vi "Get Calculated Tournament Stats.vi"(11 "Tournament Stats":T2) -> (3 "Calculated Tournament Stats":T1)   [LabVIEW 2021]
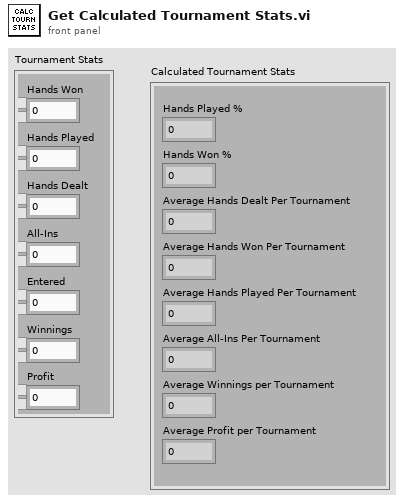
[diagram p1: front panel]
types:
  T1 = cluster{"Hands Played %":dbl, "Hands Won %":dbl, "Average Hands Dealt Per Tournament":dbl, "Average Hands Won Per Tournament":dbl, "Average Hands Played Per Tournament":dbl, "Average All-Ins Per Tournament":dbl, "Average Winnings per Tournament":dbl, "Average Profit per Tournament":dbl}
  T2 = cluster{"Hands Won":u32, "Hands Played":u32, "Hands Dealt":u32, "All-Ins":u32, "Entered":u32, "Winnings":dbl, "Profit":dbl}
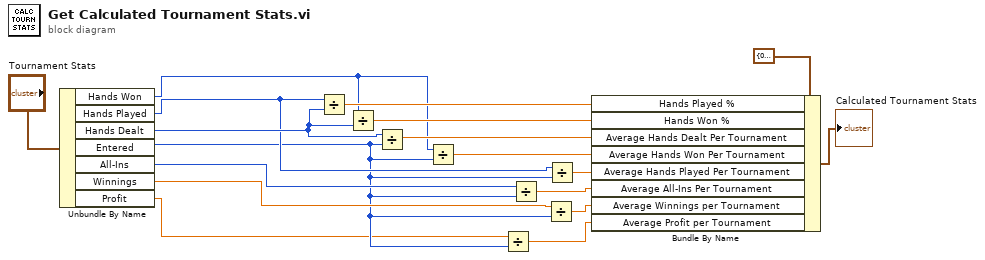
[diagram p0: block diagram]
diagram:
  n1 = Unbundle By Name("Tournament Stats") -> ("Hands Won"=w13:u32, "Hands Played"=w8:u32, "Hands Dealt"=w14:u32, "Entered"=w2:u32, "All-Ins"=w6:u32, "Winnings"=w4:dbl, "Profit"=w1:dbl)
  n2 = Divide(x=w8, y=w14) -> (x/y=w17:dbl)
  n3 = Divide(x=w13, y=w14) -> (x/y=w16:dbl)
  n4 = Divide(x=w14, y=w2) -> (x/y=w15:dbl)
  n5 = Divide(x=w13, y=w2) -> (x/y=w12:dbl)
  n6 = Divide(x=w1, y=w2) -> (x/y=w3:dbl)
  n7 = Divide(x=w6, y=w2) -> (x/y=w7:dbl)
  n8 = Divide(x=w4, y=w2) -> (x/y=w5:dbl)
  n9 = Divide(x=w8, y=w2) -> (x/y=w9:dbl)
  n10 = Bundle By Name(cluster=T1 {"Hands Played %"=0.0, "Hands Won %"=0.0, "Average Hands Dealt Per Tournament"=0.0, "Average Hands Won Per Tournament"=0.0, "Average Hands Played Per Tournament"=0.0, "Average All-Ins Per Tournament"=0.0, "Average Winnings per Tournament"=0.0, "Average Profit per Tournament"=0.0} ("Calculated Tournament Stats"), "Hands Played %"=w17, "Hands Won %"=w16, "Average Hands Dealt Per Tournament"=w15, "Average Hands Won Per Tournament"=w12, "Average Hands Played Per Tournament"=w9, "Average All-Ins Per Tournament"=w7, "Average Winnings per Tournament"=w5, "Average Profit per Tournament"=w3) -> (→"Calculated Tournament Stats":T1)
